vi "PS.Set Error Info.vi"(7 "Append Details":bool=TRUE, 8 "error in":errorcluster, 9 "Description":string, 10 "Code(0 = no change)":i32=-5303) -> (0 "error out":errorcluster)   [LabVIEW 2018]
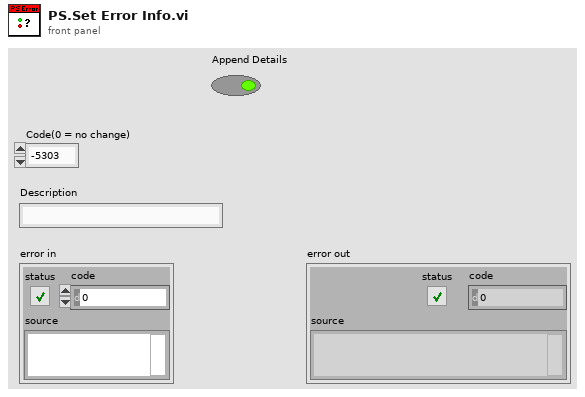
[diagram p1: front panel]
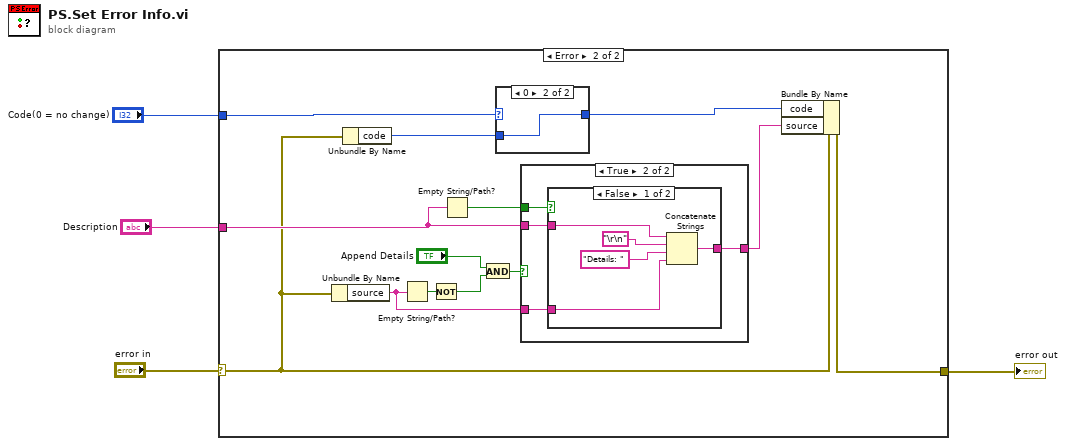
[diagram p0: block diagram]
diagram:
  n1 = case shown="Error" "error in" {
    selector: "error in" -> [w5 w6]
    tunnel: [w5 w18] -> w4
    tunnel: "Code(0 = no change)" -> [_ w12]
    tunnel: "Description" -> [_ w8]
    frame No Error {
    }
    frame Error {
      n2 = Unbundle By Name(w6) -> ("source"=w9:string)
      n3 = Unbundle By Name(w6) -> ("code"=w10:i32)
      n4 = Empty String/Path?(string/path=w9) -> (empty?=w17:bool)
      n5 = Not(x=w17) -> (.not. x?=w15:bool)
      n6 = Empty String/Path?(string/path=w8) -> (empty?=w7:bool)
      n7 = And(x="Append Details", y=w15) -> (x .and. y?=w13:bool)
      n8 = case shown="0" w12 {
        selector: w12 -> [w19 _]
        tunnel: [w19 w20] -> w11
        tunnel: w10 -> [_ w20]
        frame Default {
        }
        frame 0 {
        }
      }
      n9 = case shown="True" w13 {
        tunnel: w8 -> [w21 w30]
        tunnel: [w23 w29] -> w14
        tunnel: w9 -> [w22 w28]
        tunnel: w7 -> [w24 w27]
        frame False {
          n10 = case shown="False" w24 {
            tunnel: [w25 w26] -> w23
            tunnel: w22 -> [_ w26]
            tunnel: w21 -> [w25 _]
            frame False {
            }
            frame True {
            }
          }
        }
        frame True {
          n11 = case shown="False" w27 {
            tunnel: w30 -> [w33 _]
            tunnel: [w32 w36] -> w29
            tunnel: w28 -> [w31 w36]
            frame False {
              n12 = Concatenate Strings(w33, "\r\n", "Details: ", w31) -> (w32:string)
            }
            frame True {
            }
          }
        }
      }
      n13 = Bundle By Name(cluster=w6, "code"=w11, "source"=w14) -> (w18:errorcluster)
    }
  }
  "error out" <- w4
